vi "使用子面板.vi"() -> ()   [LabVIEW 2018]
panel:
  in  "布尔":bool
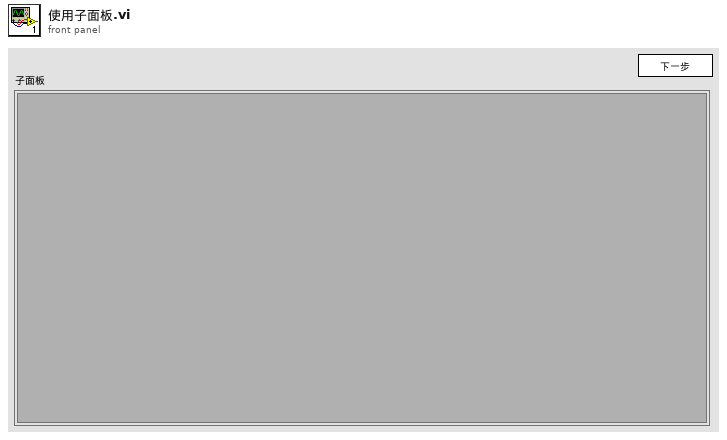
[diagram p1: front panel]
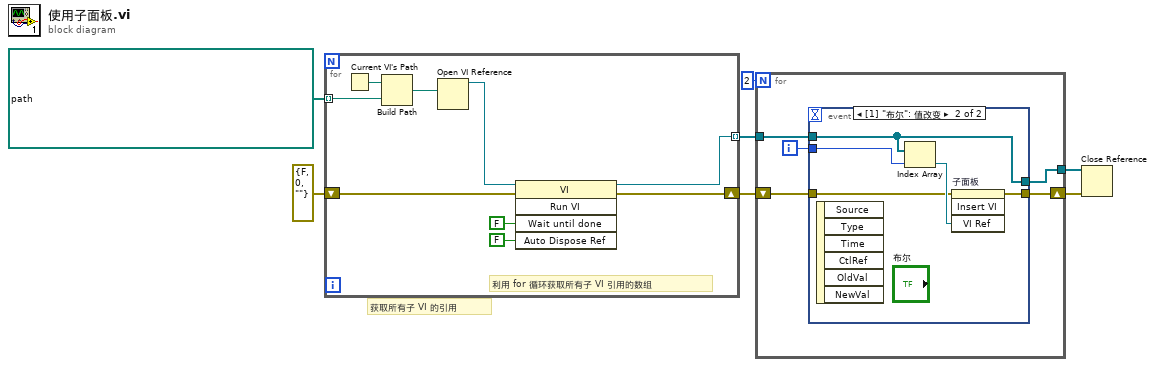
[diagram p0: block diagram]
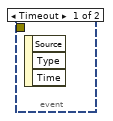
[diagram p2: hidden frame]
diagram:
  # "获取所有子 VI 的引用"
  n1 = for {
    tunnel: path[] [path "../该VI作为子面板.vi", path "../该文件同样作为子面板.vi", path "../该VI作为子面板.vi"] -> [w15] mode=indexing
    tunnel: [w10] -> w6 mode=indexing
    shift-right: [w9] -> w3
    shift-left: errorcluster {"status"=FALSE, "code"=0, "source"=""} ("error out") -> [w8]
    # "利用 for 循环获取所有子 VI 引用的数组"
    n2 = Current VI's Path() -> (path=w16:path)
    n3 = Build Path(base path=w16, name or relative path=w15) -> (appended path=w14:path)
    n4 = Open VI Reference(vi path=w14) -> (vi reference=w13:refnum<vi>)  [unwired: 5 in, 1 out]
    n5 = invoke class="VI" method="Run VI"(reference=w13, error in=w8, "Wait until done"=FALSE ("结束前等待"), "Auto Dispose Ref"=FALSE ("自动销毁引用")) -> (reference out=w10:refnum<vi>, error out=w9:errorcluster)  [unwired: 1 in, 3 out]
  }
  n6 = for {
    N: 2 -> [_]
    tunnel: w6 -> [w20]
    tunnel: [w19] -> w5
    shift-right: [w17] -> w2
    shift-left: w3 -> [w18]
    i -> [w21]
    n7 = event shown="[1] \"布尔\": 值改变" {
      selector: _ -> [_ _]
      dyn-events: _ -> [_ _]
      timeout: _ -> [_ _]
      tunnel: w20 -> [_ w24]
      tunnel: w21 -> [_ w25]
      tunnel: [_ w24] -> w19
      tunnel: w18 -> [_ w23]
      tunnel: [_ w22] -> w17
      event Timeout {
        n8 = event-data() -> ()  [unwired: 1 in, 3 out]
      }
      event "布尔": Value Change {
        n9 = event-data() -> ()  [unwired: 1 in, 6 out]
        n10 = Index Array(array=w24, index=w25) -> (element=w26:refnum<vi>)
        n11 = invoke on="子面板" class="SubPnl" method="Insert VI"(error in=w23, "VI Ref"=w26) -> (error out=w22:errorcluster)  [unwired: 2 in, 3 out]
      }
    }
  }
  n12 = Close Reference(reference=w5, error in (no error)=w2) -> ()  [unwired: 1 out]
